vi "vision_webcam_V2_external.vi"(11 "dup Message Queue 2":refnum<queue>) -> ()   [LabVIEW 2017]
uses:
  <vilib>/vision/driver/NI_Vision_Acquisition_Software.lvlib
  Globals/Global - All RT Loop Stop.vi
  <vilib>/userdefined/High Color/IMAQdx.ctl
  Globals/Global - Configuration Options.vi
  <vilib>/vision/Avi.llb/IMAQ AVI2 Refnum.ctl
  <vilib>/vision/Image Controls.llb/IMAQ Image.ctl
  <vilib>/vision/Avi.llb/IMAQ AVI2 Codec Path.ctl
  UI Error Handlers/support/Message Queue/Message Cluster.ctl
  UI Error Handlers/support/Message Queue/Message Queue.lvlib
panel:
  out "Codec Names 2":string[](array[string])
  out "Webcam":T1(plugin-control)
  out "concatenated string 4":string
  out "error out":errorcluster
  out "x-y":u32
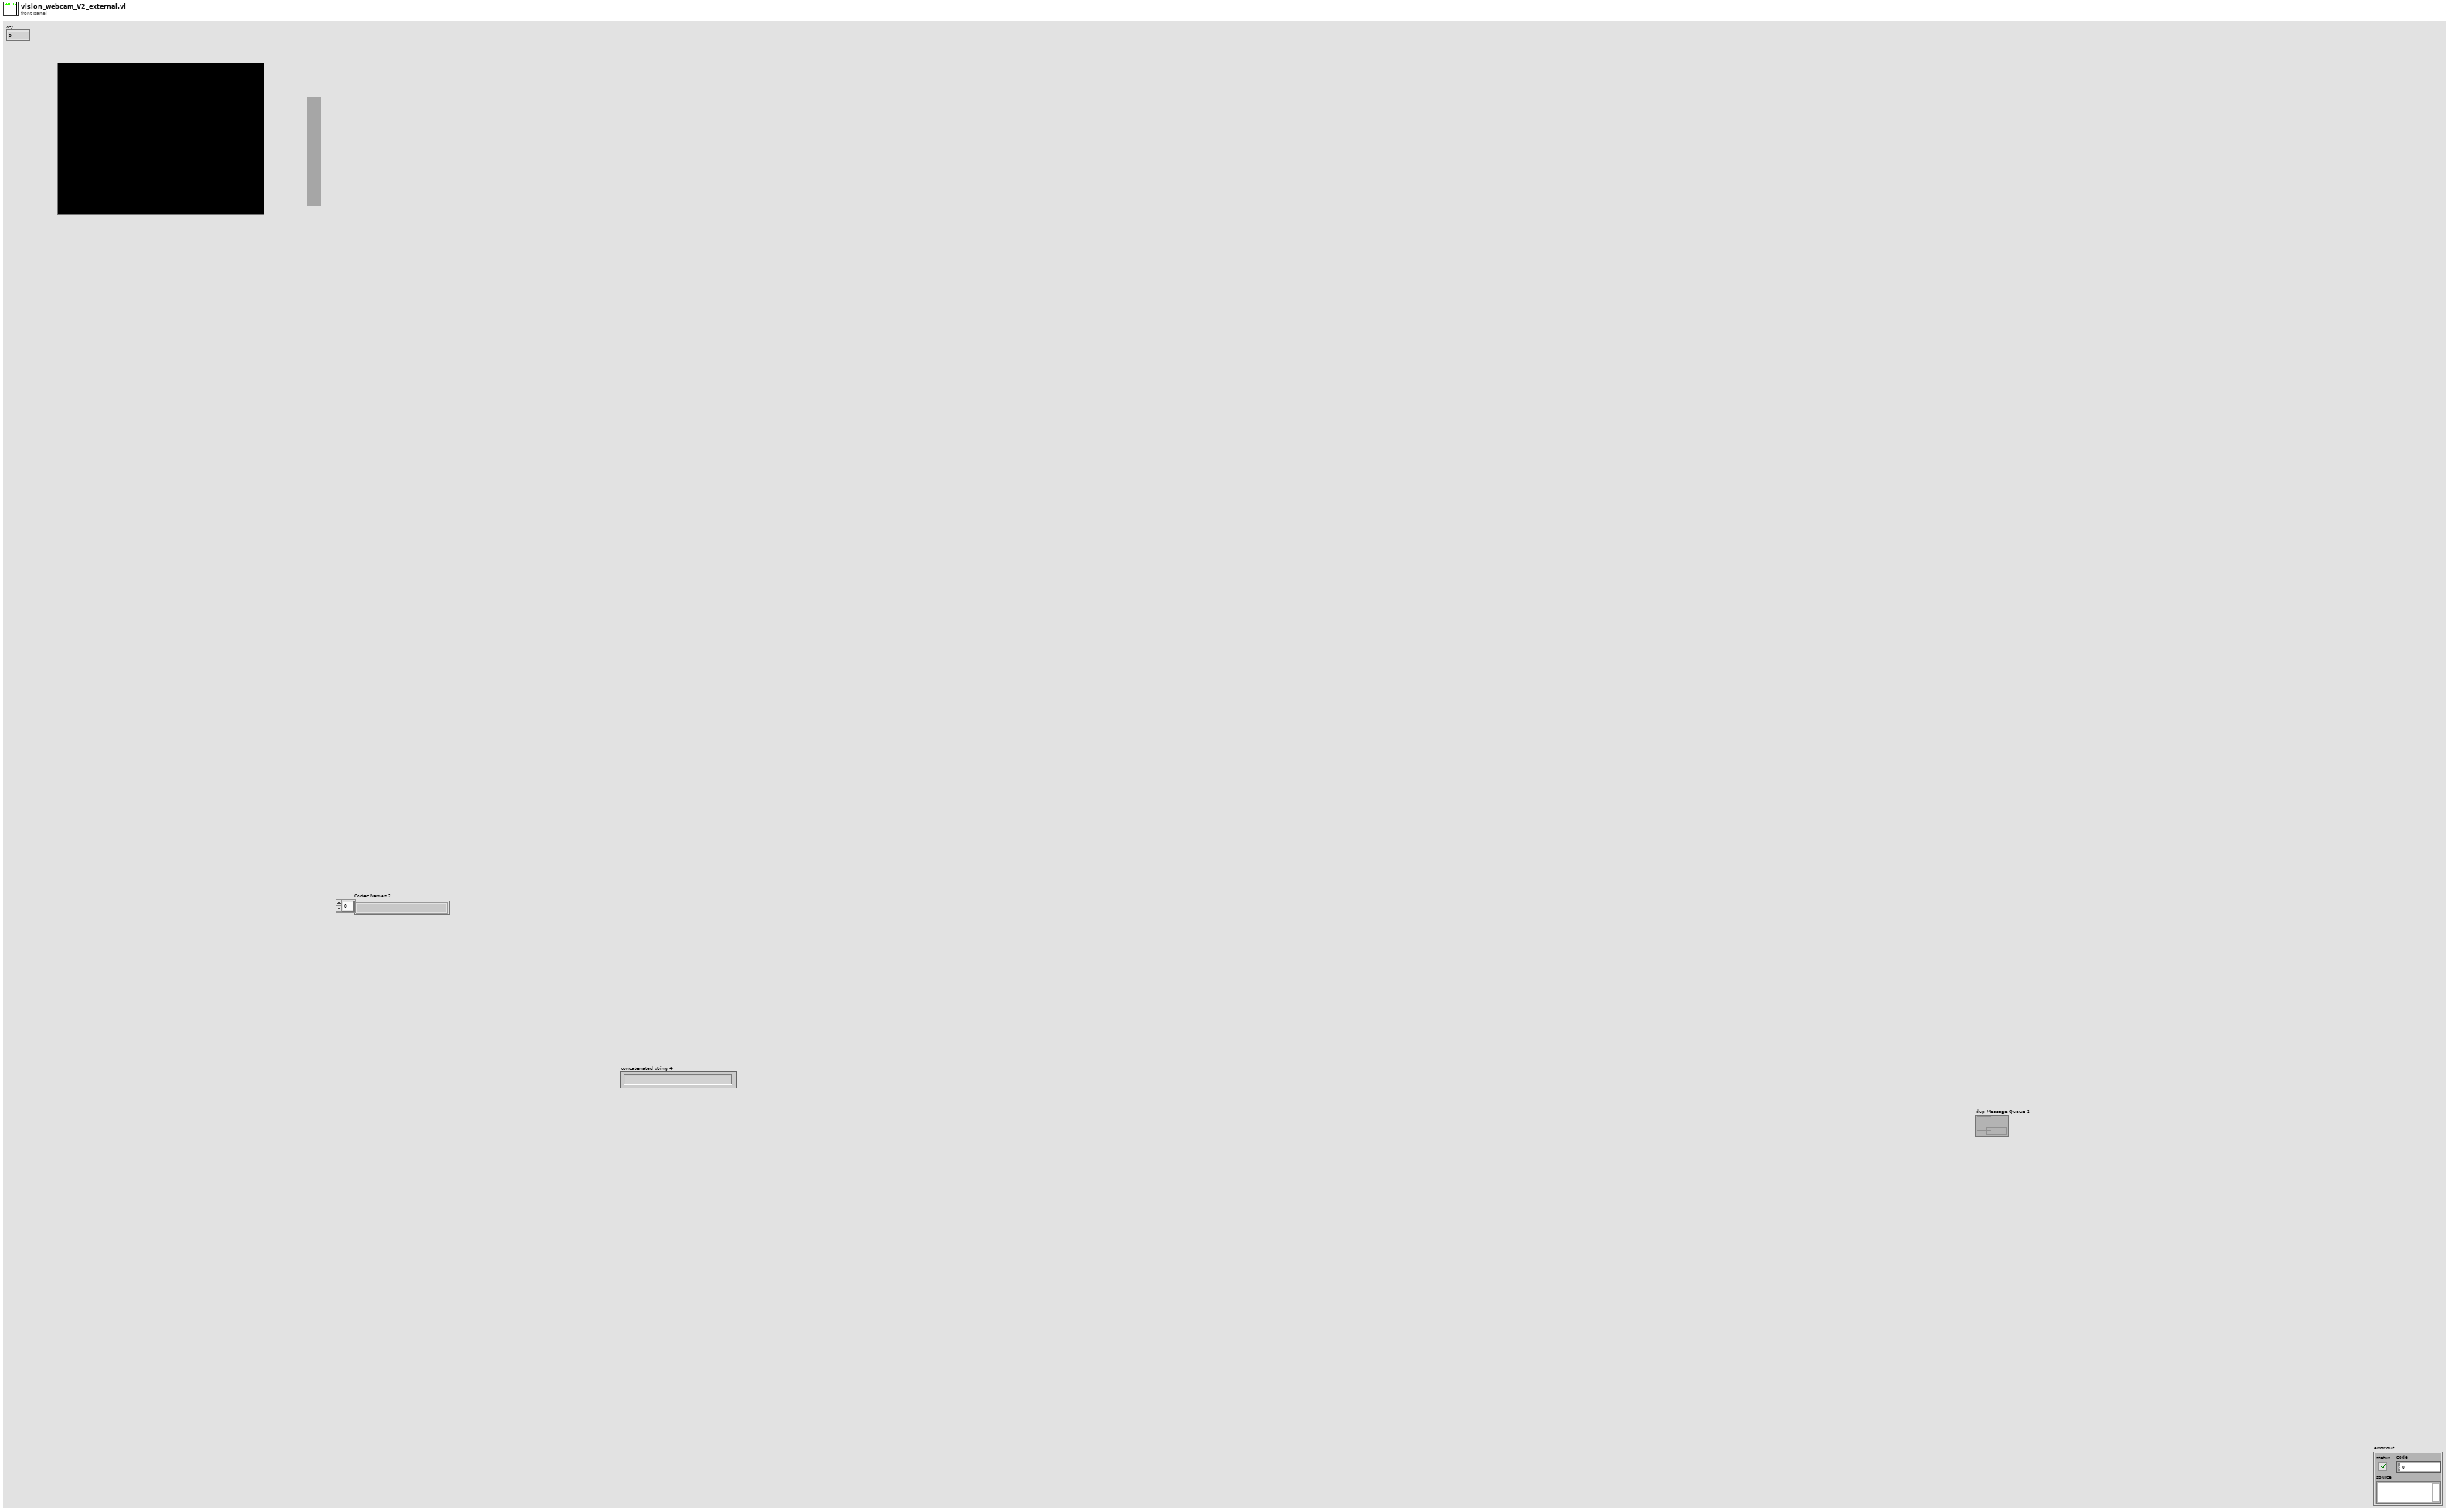
[diagram p1: front panel]
types:
  T1 = typedef "IMAQ Image.ctl" = refnum<image>
  T2 = typedef "IMAQ AVI2 Refnum.ctl" = refnum<k20>
  T3 = typedef "IMAQdx.ctl" = refnum<k21>
  T4 = typedef "Image Type" = u32
  T5 = cluster{"Tool data":cluster{"Number of teeth":sgl}, "Cutting data":cluster{"rpm":sgl}, "Limits":cluster{"Magnitude threshold":sgl, "Tolerance":sgl}, "G1 status":cluster{"G1 trigger":bool}}
  T6 = typedef "IMAQ AVI2 Codec Path.ctl" = u32
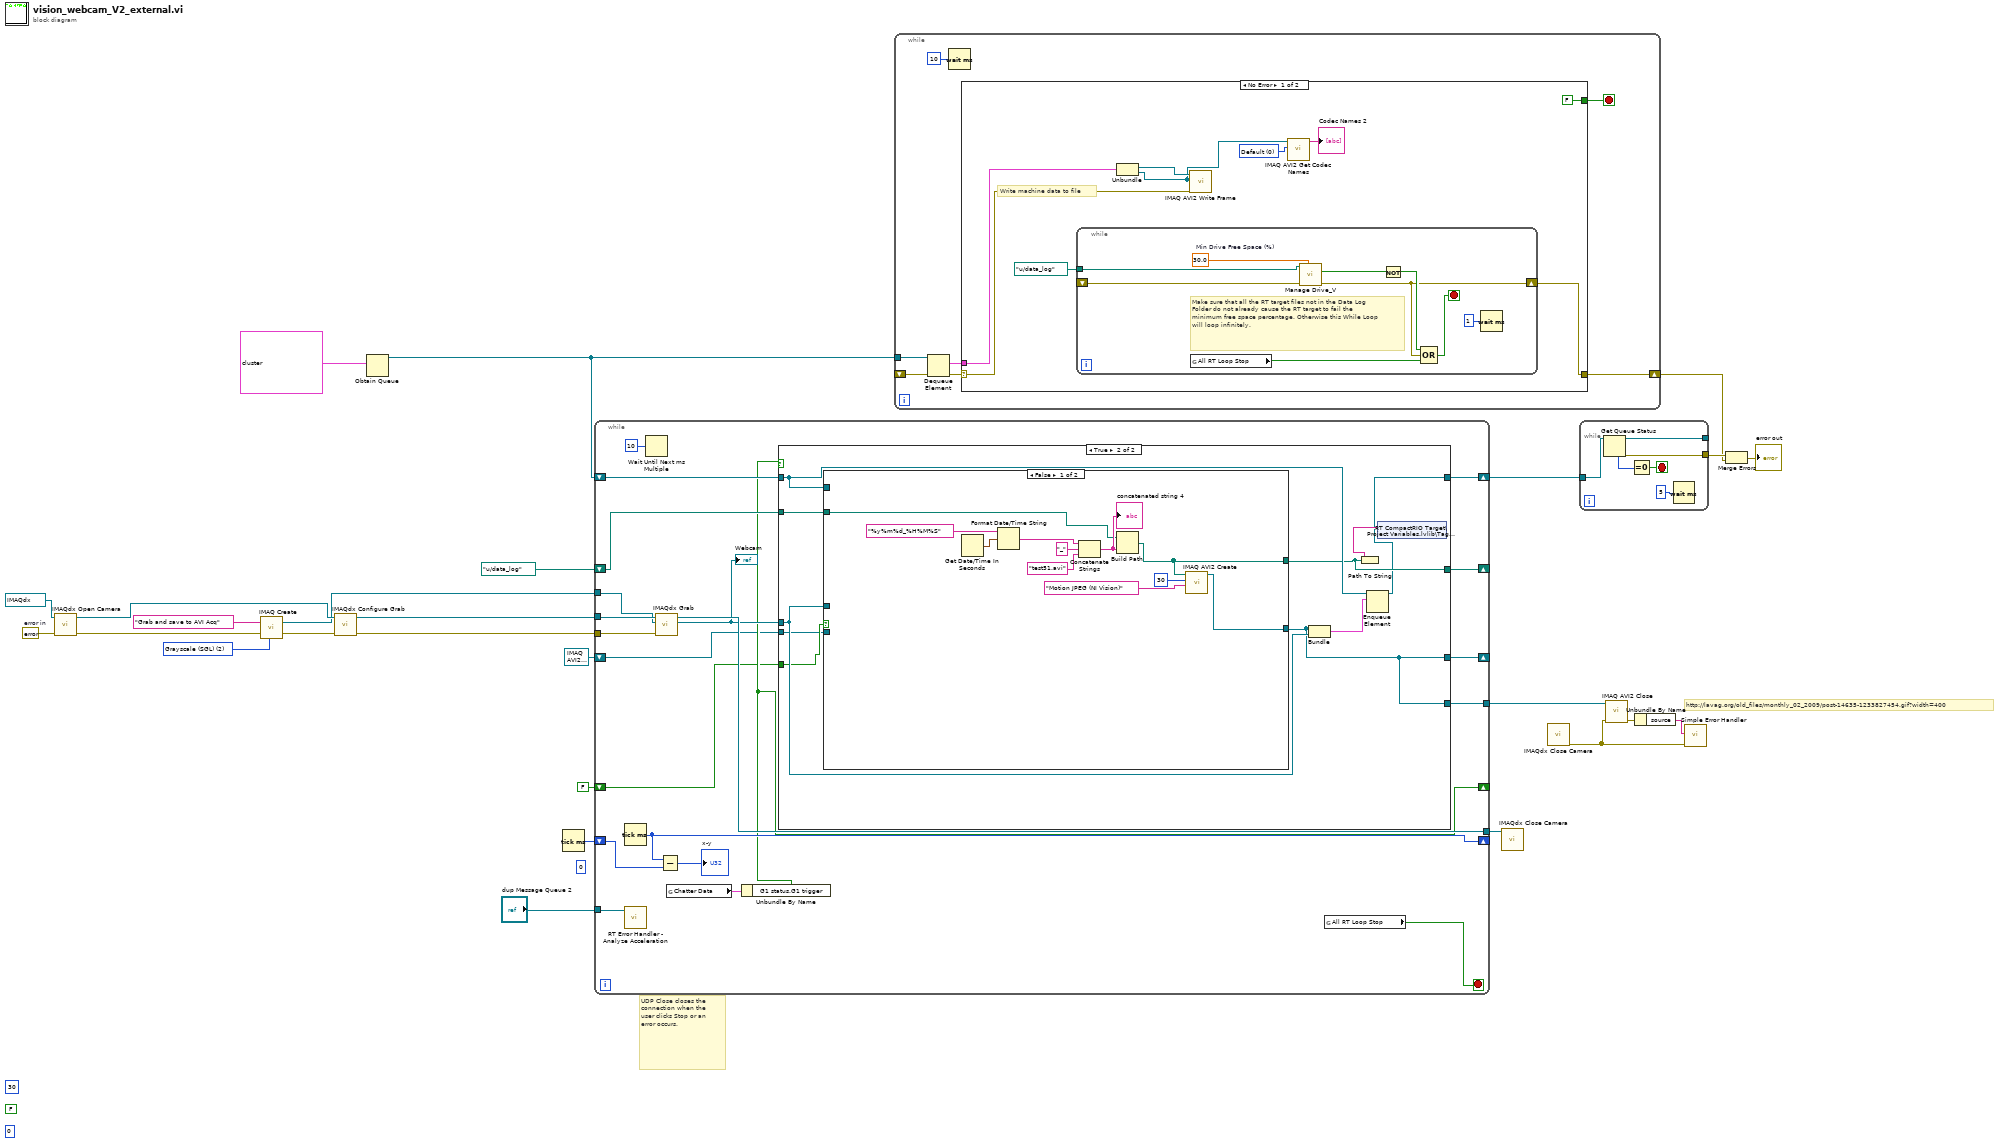
[diagram p0: block diagram]
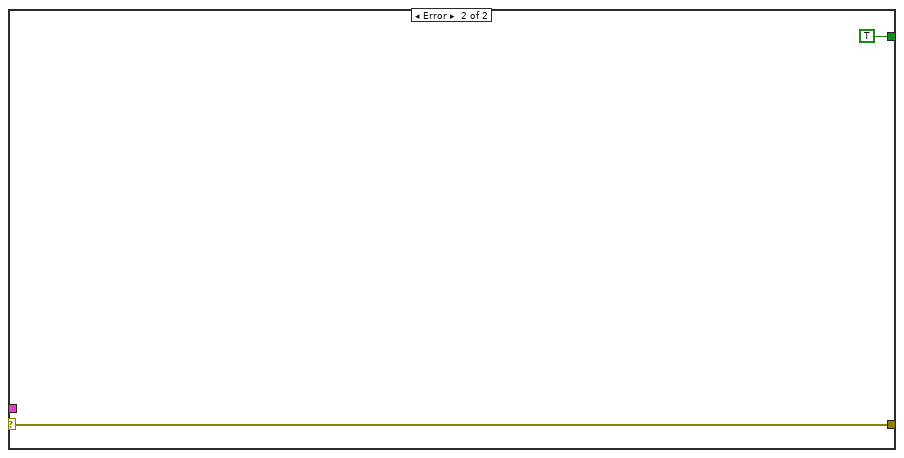
[diagram p2: hidden frame]
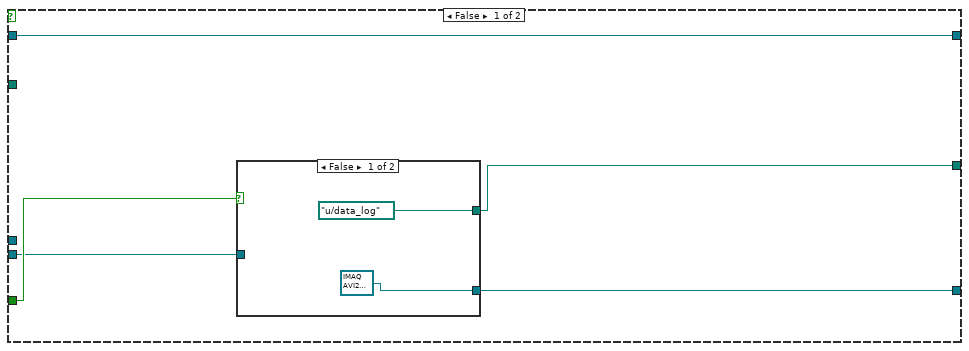
[diagram p3: hidden frame]
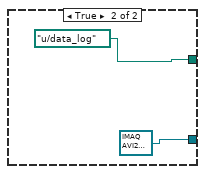
[diagram p4: hidden frame]
diagram:
  (unwired) 0
  w16 = T4 2 items=["Grayscale (U8)", "Grayscale (I16)", "Grayscale (SGL)", "Complex (CSG)", "RGB (U32)", "HSL (U32)", "RGB (U64)", "Grayscale (U16)"] ("Image Type")
  (unwired) u32 30 ("Frames Per Second")
  w17 = errorcluster {"status"=FALSE, "code"=0, "source"=""}  # error in
  (unwired) i16 0 ("A(I16) 11")
  (unwired) FALSE
  # "http://lavag.org/old_files/monthly_02_2009/post-14635-1233827454.gif?width=400"
  # "UDP Close closes the connection when the user clicks Stop or an error occurs."
  n1 = call <vilib>:"IMAQdx Open Camera.vi"("error in"=w17, "Session In"=T3 "cam1") -> ("error out"=w15:errorcluster, "Session Out"=w19:T3)  [unwired: 8 in]
  n2 = call "IMAQ Create"("Image Name"="Grab and save to AVI Acq", "Image Type"=w16, "error in (no error)"=w15) -> ("New Image"=w12:T1, "error out"=w11:errorcluster)  [unwired: 2 in]
  n3 = call <vilib>:"IMAQdx Configure Grab.vi"("error in"=w11, "Session In"=w19) -> ("error out"=w10:errorcluster, "Session Out"=w13:T3)  [unwired: 8 in]
  n4 = Obtain Queue(element data type=cluster{"AVI Refnum 2":T2, "Image Out 2":T1} {"AVI Refnum 2"=refnum, "Image Out 2"=refnum}) -> (queue out=w24:refnum<queue>)  [unwired: 4 in, 2 out]
  n5 = Tick Count (ms)() -> (millisecond timer value=w20:u32)
  n6 = while {
    shift-right: [w46] -> w26
    shift-left: w24 -> [w47]
    tunnel: "dup Message Queue 2" -> [w45]
    shift-right: [w41] -> _
    shift-left: w20 -> [w42]
    tunnel: w13 -> [w40]
    tunnel: w12 -> [w39]
    tunnel: w10 -> [w38]
    tunnel: [w37] -> w9
    shift-right: [w32] -> _
    shift-left: path "u:/data_log" ("AVI Path") -> [w33]
    shift-right: [w31] -> _
    shift-left: FALSE ("G1 trigger") -> [w30]
    shift-right: [w28] -> _
    shift-left: T2 refnum ("AVI Refnum") -> [w29]
    tunnel: [w27] -> w1
    stop <- w35 stop-if-true
    n7 = Tick Count (ms)() -> (millisecond timer value=w41:u32)
    n8 = call "RT Error Handler - Analyze Acceleration.vi"("Message Queue"=w45) -> ()  [unwired: 10 in, 1 out]
    n9 = Wait Until Next ms Multiple(millisecond multiple=u32 10) -> ()  [unwired: 1 out]
    n10 = call <vilib>:"IMAQdx Grab.vi"("error in"=w38, "Image In"=w39, "Session In"=w40) -> ("Image Out"=w34:T1, "Session Out"=w37:T3)  [unwired: 5 in, 2 out]
    "Webcam" <- w34
    n11 = Subtract(x=w41, y=w42) -> (x-y=→"x-y":u32)
    n12 = global read "Global - Configuration Options.vi" "Chatter Data"() -> (w44:T5)
    n13 = Unbundle By Name(w44) -> ("G1 status.G1 trigger"=w31:bool)
    n14 = case shown="True" w31 {
      tunnel: w47 -> [w52 w65]
      tunnel: [w52 w60] -> w46
      tunnel: w34 -> [_ w66]
      tunnel: w33 -> [_ w63]
      tunnel: [w51 w62] -> w32
      tunnel: w30 -> [w50 w61]
      tunnel: w29 -> [w49 w58]
      tunnel: [w48 w57] -> w28
      tunnel: [_ w57] -> w27
      frame False {
        n15 = case shown="False" w50 {
          tunnel: [path "u:/data_log" ("AVI Path") path "u:/data_log" ("AVI Path")] -> w51
          tunnel: w49 -> [_ _]
          tunnel: [T2 refnum ("AVI Refnum") T2 refnum ("AVI Refnum")] -> w48
          frame False {
          }
          frame True {
          }
        }
      }
      frame True {
        n16 = case shown="False" w61 {
          tunnel: w66 -> [_ _]
          tunnel: w65 -> [_ _]
          tunnel: [w69 w79] -> w62
          tunnel: w63 -> [w68 w79]
          tunnel: [w67 w78] -> w57
          tunnel: w58 -> [_ w78]
          frame False {
            n17 = Get Date/Time In Seconds() -> (seconds since 1Jan1904=w75:timestamp)
            n18 = Format Date/Time String(time format string (%c)="%y%m%d_%H%M%S", seconds (now)=w75) -> (date/time string=w76:string)  [unwired: 1 out]
            n19 = Concatenate Strings(w76, "_" ("string"), "test51.avi" ("name or relative path")) -> (w77:string)
            "concatenated string 4" <- w77
            n20 = Build Path(base path=w68, name or relative path=w77) -> (appended path=w69:path)
            n21 = call "IMAQ AVI2 Create"("Codec"="Motion JPEG (NI Vision)", "Frames Per Second"=u32 30, "AVI Path"=w69) -> ("AVI Refnum"=w67:T2)  [unwired: 7 in, 1 out]
          }
          frame True {
          }
        }
        n22 = Bundle("AVI Refnum"=w57, "Image Out"=w66) -> (w59:cluster{"AVI Refnum":T2, "Image Out":T1})  [unwired: 1 in]
        n23 = Path To String(path=w62) -> (string=w64:string)
        n24 = Enqueue Element(queue=w65, element=w59) -> (queue out=w60:refnum<queue>)  [unwired: 2 in, 2 out]
        n25 = shared-variable "RT CompactRIO Target\\Project Variables.lvlib\\Tag Video"(w64) -> ()  [unwired: 1 in, 1 out]
      }
    }
    n26 = global read "Global - All RT Loop Stop.vi" "All RT Loop Stop"() -> (w35:bool)
  }
  n27 = while {
    tunnel: w24 -> [w86]
    shift-right: [w82] -> w23
    shift-left: _ -> [w85]
    stop <- w83 stop-if-true
    n28 = Dequeue Element(queue=w86, error in (no error)=w85) -> (element=w81:cluster{"AVI Refnum 2":T2, "Image Out 2":T1}, error out=w84:errorcluster)  [unwired: 1 in, 2 out]
    n29 = Wait (ms)(milliseconds to wait=u32 10) -> ()  [unwired: 1 out]
    n30 = case shown="No Error" w84 {
      selector: w84 -> [w94 w105]
      tunnel: [FALSE TRUE] -> w83
      tunnel: [w92 w105] -> w82
      tunnel: w81 -> [w91 _]
      frame No Error {
        w89 = T6 0 items=["Default", "System", "Built in Vision"] ("Codec Source")
        # "Write machine data to file"
        n31 = while {
          shift-right: [w99] -> w92
          shift-left: _ -> [w100]
          tunnel: path "u:/data_log" ("AVI Path") -> [w97]
          stop <- w104 stop-if-true
          w98 = 30.0  # Min Drive Free Space (%)
          # "Make sure that all the RT target files not in the Data Log Folder do not already cause the RT target to fail the minimum free space percentage. Otherwise this While Loop will loop infinitely."
          n32 = global read "Global - All RT Loop Stop.vi" "All RT Loop Stop"() -> (w101:bool)
          n33 = call "Manage Drive_V.vi"("Min Drive Free Space (%)"=w98, "error in"=w100, "Data Folder"=w97) -> ("error out"=w99:errorcluster, "Drive Space Below Limit"=w96:bool)  [unwired: 6 in, 1 out]
          n34 = Not(x=w96) -> (.not. x?=w103:bool)
          n35 = Compound Arithmetic op=OR(w103, w99, w101) -> (w104:bool)
          n36 = Wait (ms)(milliseconds to wait=u32 1) -> ()  [unwired: 1 out]
        }
        n37 = Unbundle(w91) -> ("AVI Refnum 2"=w90:T2, "Image Out 2"=w87:T1)
        n38 = call "IMAQ AVI2 Write Frame"("error in (no error)"=w94, "Image"=w87, "AVI Refnum"=w90) -> ()  [unwired: 6 in, 3 out]
        n39 = call "IMAQ AVI2 Get Codec Names"("Codec Source"=w89, "Image"=w87) -> ("Codec Names"=→"Codec Names 2":string[])  [unwired: 8 in, 1 out]
      }
      frame Error {
      }
    }
  }
  n40 = call <vilib>:"IMAQdx Close Camera.vi"("Session In"=w9) -> ()  [unwired: 10 in, 1 out]
  n41 = call <vilib>:"IMAQdx Close Camera.vi"() -> ("error out"=w3:errorcluster)  [unwired: 11 in]
  n42 = while {
    tunnel: [w111] -> w25
    tunnel: [w109] -> _
    tunnel: w26 -> [w107]
    stop <- w110 stop-if-true
    n43 = Get Queue Status(queue=w107) -> (queue out=w109:refnum<queue>, error out=w111:errorcluster, # elements in queue=w108:i32)  [unwired: 2 in, 5 out]
    n44 = Equal To 0?(x=w108) -> (x = 0?=w110:bool)
    n45 = Wait (ms)(milliseconds to wait=u32 5) -> ()  [unwired: 1 out]
  }
  n46 = call "IMAQ AVI2 Close"("error in (no error)"=w3, "AVI Refnum"=w1) -> ("error out"=w4:errorcluster)  [unwired: 9 in]
  n47 = Unbundle By Name(w4) -> ("source"=w2:string)
  n48 = call <vilib>:"Simple Error Handler.vi"("error source (\" \")"=w2, "error in (no error)"=w3) -> ()  [unwired: 3 in, 5 out]
  n49 = Merge Errors(w25, w23) -> (→"error out":errorcluster)
